vi "mass Cleanup (Folder).vi"() -> ()   [LabVIEW 2020]
uses:
  <vilib>/Utility/traverseref.llb/TRef TravTarget.ctl
  <vilib>/Utility/traverseref.llb/VI Scripting - Traverse.lvlib
panel:
  in  "Source folder":path
  in  "scan folders":bool
  in  "Show FP (F)":bool=TRUE
  out "Slide":u8(slide) scale=0.0..100.0
  out "error":i32
  out "relinked":i32
  in  "Arrange":bool
  in  "FP (T)":bool=TRUE
  out "error out":errorcluster
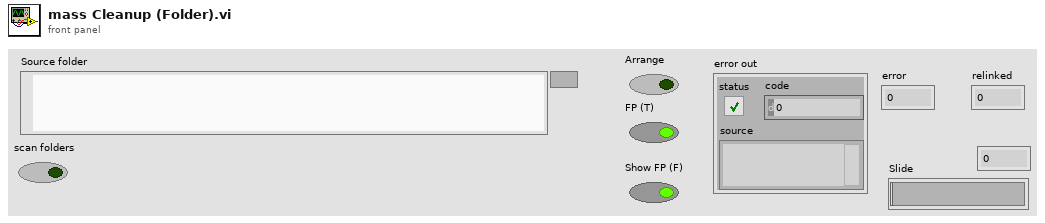
[diagram p1: front panel]
types:
  T1 = typedef "TRef TravTarget.ctl" = enum16{"FP", "BD", "Other"}
  T2 = enum32{"invalid VI type", "Standard VI", "Control VI", "Global VI", "Polymorphic VI", "Configuration VI", "SubSystem", "Facade VI", "Method VI", "Statechart Diagram VI"}
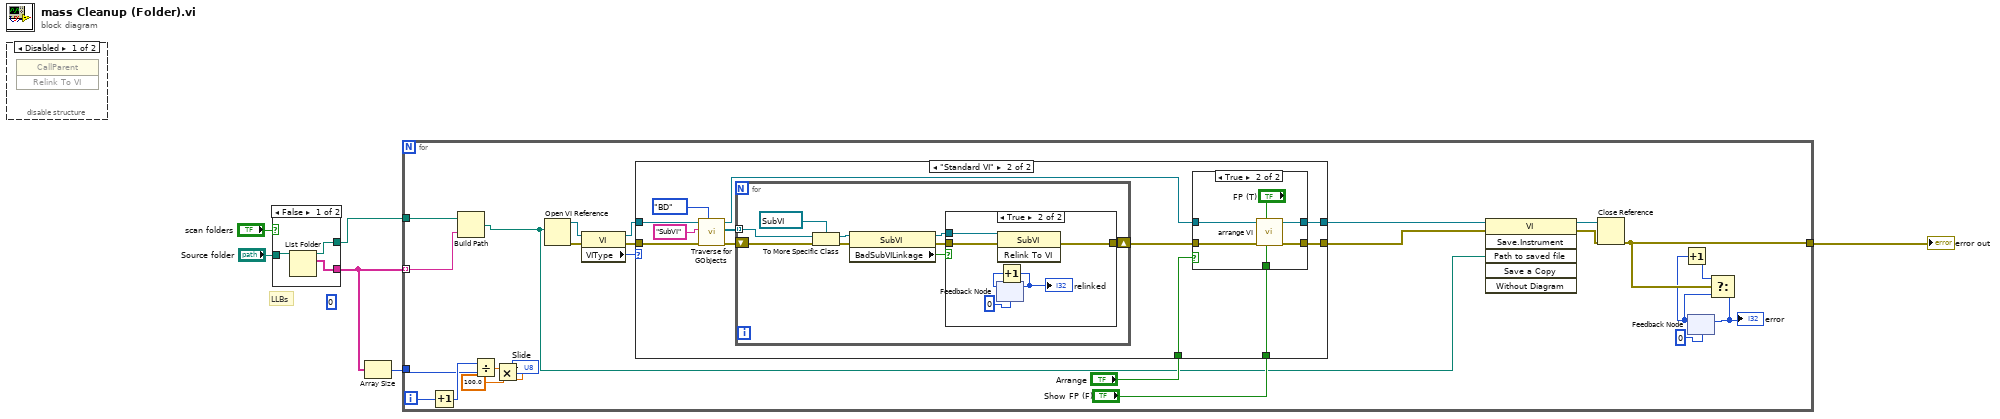
[diagram p0: block diagram]
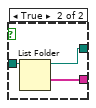
[diagram p2: hidden frame]
diagram:
  (unwired) 0
  # "LLBs"
  n1 = disable-structure shown="Disabled" {
    frame Disabled {
      n2 = invoke class="CallParent" method="Relink To VI"() -> ()  [unwired: 3 in, 3 out]
    }
    frame Enabled {
    }
  }
  n3 = case shown="False" "scan folders" {
    tunnel: "Source folder" -> [w9 w12]
    tunnel: [w8 w11] -> w2
    tunnel: [w7 w10] -> w1
    frame False {
      n4 = List Folder(path=w9) -> (path out=w8:path, filenames=w7:string[])  [unwired: 3 in, 2 out]
    }
    frame True {
      n5 = List Folder(path=w12) -> (path out=w11:path, folder names=w10:string[])  [unwired: 3 in, 2 out]
    }
  }
  n6 = Array Size(array=w1) -> (size(s)=w5:i32)
  n7 = for {
    tunnel: [w28] -> w6
    tunnel: w5 -> [w23]
    tunnel: w2 -> [w15]
    tunnel: w1 -> [w14] mode=indexing
    i -> [w30]
    n8 = Increment(x=w30) -> (x+1=w24:i32)
    n9 = Build Path(base path=w15, name or relative path=w14) -> (appended path=w13:path)
    n10 = Divide(x=w24, y=w23) -> (x/y=w22:dbl)
    n11 = Multiply(x=w22, y=100.0) -> (x*y=→"Slide":dbl)
    n12 = Open VI Reference(vi path=w13) -> (vi reference=w37:refnum<vi>, error out=w35:errorcluster)  [unwired: 5 in]
    n13 = property class="VI"(reference=w37, error in=w35) -> (reference out=w36:refnum<vi>, error out=w34:errorcluster, "VIType"=w33:T2)
    n14 = case shown="\"Standard VI\"" w33 {
      tunnel: [w39 w40] -> w16
      tunnel: w36 -> [w38 w47]
      tunnel: w34 -> [w39 w46]
      tunnel: "Arrange" -> [_ w45]
      tunnel: "Show FP (F)" -> [_ w42]
      tunnel: [w38 w41] -> w17
      frame "invalid VI type", Default {
      }
      frame "Standard VI" {
        n15 = call <vilib>:"Traverse for GObjects.vi"("Traverse Target"=TRef_TravTarget."BD", "error in (no error)"=w46, "Class Name"="SubVI", "VI Refnum"=w47) -> ("error out"=w49:errorcluster, "References"=w50:refnum<vi>[], "dup VI Refnum"=w43:refnum<vi>)  [unwired: 4 in, 1 out]
        n16 = for {
          tunnel: w50 -> [w66] mode=indexing
          shift-right: [w60] -> w44
          shift-left: w49 -> [w65]
          n17 = To More Specific Class(target class=refnum<vi> refnum ("reference"), reference=w66, error in=w65) -> (specific class reference=w61:refnum<vi>, error out=w68:errorcluster)
          n18 = property class="SubVI"(reference=w61, error in=w68) -> (reference out=w62:refnum<vi>, error out=w63:errorcluster, "BadSubVILinkage"=w64:bool)
          n19 = case shown="True" w64 {
            tunnel: w63 -> [w69 w73]
            tunnel: w62 -> [_ w74]
            tunnel: [w69 w75] -> w60
            frame False {
            }
            frame True {
              n20 = feedback #1(0) -> (w71:i32)
              n21 = invoke class="SubVI" method="Relink To VI"(reference=w74, error in=w73) -> (error out=w75:errorcluster)  [unwired: 1 in, 2 out]
              n22 = Increment(x=w71) -> (x+1=w70:i32)
              "relinked" <- w70
              n23 = feedback-in #1(w70) -> ()
            }
          }
        }
        n24 = case shown="True" w45 {
          tunnel: w44 -> [w52 w59]
          tunnel: [w52 w58] -> w40
          tunnel: w43 -> [w53 w57]
          tunnel: [w53 w56] -> w41
          tunnel: w42 -> [_ w54]
          frame False {
          }
          frame True {
            n25 = call "arrange VI.vi"("Show FP (F)"=w54, "FP (T)"="FP (T)", "error in"=w59, "VI in"=w57) -> ("error out"=w58:errorcluster, "VI out"=w56:refnum<vi>)  [unwired: 6 in]
          }
        }
      }
    }
    n26 = invoke class="VI" method="Save.Instrument"(reference=w17, error in=w16, "Path to saved file"=w13) -> (reference out=w31:refnum<vi>, error out=w32:errorcluster)  [unwired: 3 in, 4 out]
    n27 = Close Reference(reference=w31, error in (no error)=w32) -> (error out=w28:errorcluster)
    n28 = feedback #2(0) -> (w27:i32)
    n29 = Increment(x=w27) -> (x+1=w26:i32)
    n30 = Select(t=w26, s=w28, f=w27) -> (s? t:f=w25:i32)
    "error" <- w25
    n31 = feedback-in #2(w25) -> ()
  }
  "error out" <- w6
